vi "Climb_Globals.vi"() -> ()   [LabVIEW 2019]
panel:
  in  "Climb_Transverse":string="Climb_Transverse"
  in  "Climb_Elevator_Left":string="Climb_Elevator_Left"
  in  "Climb_Elevator_Right":string="Climb_Elevator_Right"
  in  "Climb_Pivot":string="Climb_Pivot"
  in  "Climb_Execute_Ref":string="ClimbExecuteRef"
  in  "Climb_Set_Ref":string="ClimbSetRef"
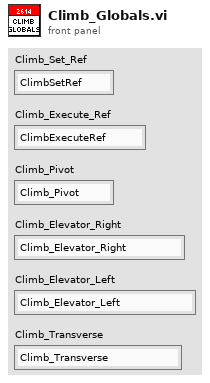
[diagram p1: front panel]
diagram:
